vi "about.vi"   [LabVIEW 2015]
uses:
  ESLSCDLL.dll
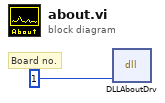
[diagram p0: block diagram]
diagram:
  # "Board no."
  n1 = dll-call lib="C:/ENTW/PCIE/64bit/lv64/1cam/board.vis/ESLSCDLL.dll" fn="DLLAboutDrv"("drv"=u32 1) -> ()  [unwired: 5 in, 2 out]
